vi "Documentation Panel.vi"() -> ()   [LabVIEW 2019, in "Panther Dashboard.lvlib"]
uses:
  Panther Dashboard.lvlib
panel:
  in  "Edit Module Description":bool caption="Module Description- Edit"
  in  "Module Description":string
  in  "Edit VI":bool caption="Event Connector Pane- Edit"
  out "Event Connector Pane":picture
  in  "Event Description":string
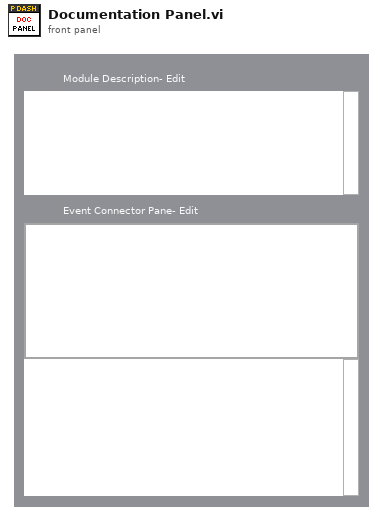
[diagram p1: front panel]
types:
  T1 = typedef "Panther Dashboard.lvlib/Broadcast Events--cluster.ctl" = cluster{"Module Did Init":refnum<user-event>, "Status Updated":refnum<user-event>, "Error Reported":refnum<user-event>, "Module Did Stop":refnum<user-event>, "Update Module Execution Status":refnum<user-event>, "References Updated":refnum<user-event>, "Projects Updated":refnum<user-event>, "Targets Updated":refnum<user-event>, "Progress updated":refnum<user-event>, "Scale Updated":refnum<user-event>, "Connector Pane Updated":refnum<user-event>, "Documentation Updated":refnum<user-event>, "Module Type Updated":refnum<user-event>, "Theme Updated":refnum<user-event>, "Panel Position Updated":refnum<user-event>}
  T2 = enum8{"Enabled", "Disabled", "Disabled and Grayed Out"}
  T3 = typedef "Panther Dashboard.lvlib/Documentation--cluster.ctl" = cluster{"Module Description":string, "Event Description":string}
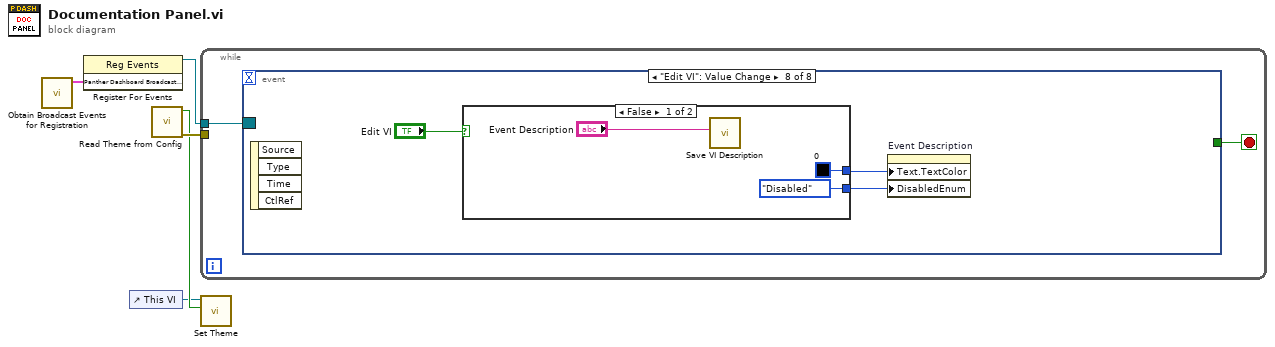
[diagram p0: block diagram]
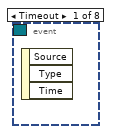
[diagram p2: hidden frame]
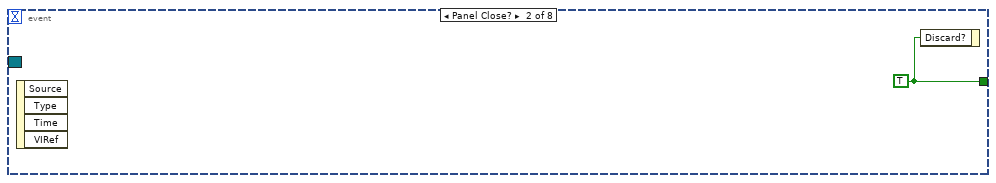
[diagram p3: hidden frame]
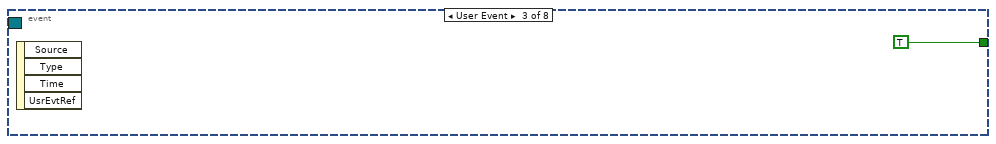
[diagram p4: hidden frame]
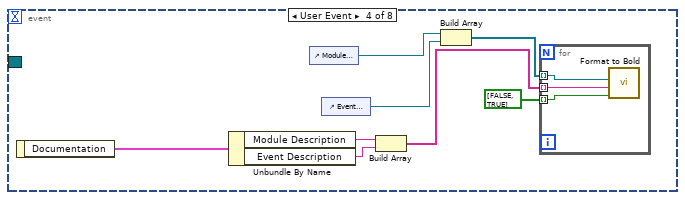
[diagram p5: hidden frame]
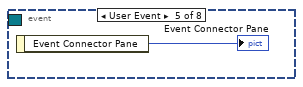
[diagram p6: hidden frame]
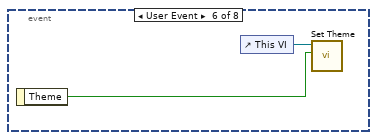
[diagram p7: hidden frame]
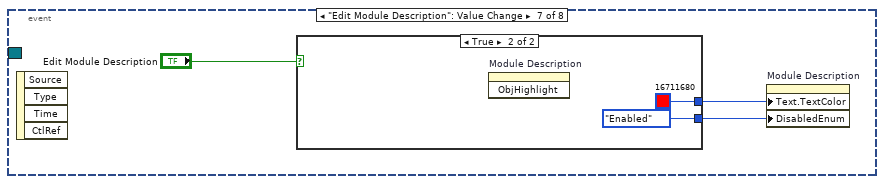
[diagram p8: hidden frame]
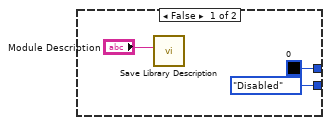
[diagram p9: hidden frame]
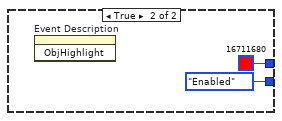
[diagram p10: hidden frame]
diagram:
  n1 = call "Obtain Broadcast Events for Registration.vi"() -> ("Panther Dashboard Broadcast Events"=w4:T1)  [unwired: 9 in, 2 out]
  n2 = register-events(w4) -> (reference out=w3:refnum<event-registration>)  [unwired: 2 in, 1 out]
  n3 = control-ref of="This VI"() -> (w1:refnum<vi>)
  n4 = call "Read Theme from Config.vi"() -> ("error out"=w5:errorcluster, "Theme"=w2:bool)  [unwired: 10 in]
  n5 = while {
    tunnel: w3 -> [w7]
    tunnel: w5 -> [_]
    stop <- w6 stop-if-true
    n6 = event shown="[7] \"Edit VI\": Value Change" {
      selector: w7 -> [_ _ _ _ _ _ _ _]
      dyn-events: _ -> [_ _ _ _ _ _ _ _]
      timeout: _ -> [_ _ _ _ _ _ _ _]
      tunnel: [_ w8 TRUE ("Discard?") _ _ _ _ _] -> w6
      event Timeout {
        n7 = event-data() -> ()  [unwired: 1 in, 3 out]
      }
      event Panel Close? {
        w8 = TRUE ("Discard?")
        n8 = event-data() -> ()  [unwired: 1 in, 4 out]
        n9 = event-data("Discard?"=w8) -> ()  [unwired: 1 in, 1 out]
      }
      event User Event {
        n10 = event-data() -> ()  [unwired: 1 in, 4 out]
      }
      event User Event {
        n11 = event-data() -> ("Documentation"=w10:T3)  [unwired: 1 in]
        n12 = Unbundle By Name(w10) -> ("Module Description"=w12:string, "Event Description"=w13:string)
        n13 = control-ref of="Module Description"() -> (w14:refnum<vi>)
        n14 = control-ref of="Event Description"() -> (w15:refnum<vi>)
        n15 = Build Array(w12, w13) -> (w17:string[])
        n16 = Build Array(w14, w15) -> (w16:refnum<vi>[])
        n17 = for {
          tunnel: w16 -> [w20] mode=indexing
          tunnel: w17 -> [w19] mode=indexing
          tunnel: bool[] [FALSE, TRUE] ("Adjust Height?") -> [w18] mode=indexing
          n18 = call "Format to Bold.vi"("Adjust Height?"=w18, "String Value"=w19, "String Ref"=w20) -> ()  [unwired: 9 in]
        }
      }
      event User Event {
        n19 = event-data() -> ("Event Connector Pane"=→"Event Connector Pane":picture)  [unwired: 1 in]
      }
      event User Event {
        n20 = event-data() -> ("Theme"=w22:bool)  [unwired: 1 in]
        n21 = control-ref of="This VI"() -> (w23:refnum<vi>)
        n22 = call "Set Theme.vi"("Dark?"=w22, "VI in"=w23) -> ()  [unwired: 10 in]
      }
      event "Edit Module Description": Value Change {
        n23 = event-data() -> ()  [unwired: 1 in, 4 out]
        n24 = case shown="True" "Edit Module Description" {
          tunnel: [u32 0 u32 16711680] -> w25
          tunnel: [T2."Disabled" ("Disabled") T2."Enabled" ("Disabled")] -> w24
          frame False {
            n25 = call "Save Library Description.vi"("Library Description"="Module Description") -> ()  [unwired: 10 in, 1 out]
          }
          frame True {
            n26 = invoke on="Module Description" class="Str" method="ObjHighlight"() -> ()  [unwired: 3 in, 3 out]
          }
        }
        n27 = property on="Module Description" class="Str"("Text.TextColor"=w25, "DisabledEnum"=w24) -> ()  [unwired: 2 in, 2 out]
      }
      event "Edit VI": Value Change {
        n28 = event-data() -> ()  [unwired: 1 in, 4 out]
        n29 = case shown="False" "Edit VI" {
          tunnel: [u32 0 u32 16711680] -> w33
          tunnel: [T2."Disabled" ("Disabled") T2."Enabled" ("Disabled")] -> w32
          frame False {
            n30 = call "Save VI Description.vi"("VI Description"="Event Description") -> ()  [unwired: 10 in, 1 out]
          }
          frame True {
            n31 = invoke on="Event Description" class="Str" method="ObjHighlight"() -> ()  [unwired: 3 in, 3 out]
          }
        }
        n32 = property on="Event Description" class="Str"("Text.TextColor"=w33, "DisabledEnum"=w32) -> ()  [unwired: 2 in, 2 out]
      }
    }
  }
  n33 = call "Set Theme.vi"("Dark?"=w2, "VI in"=w1) -> ()  [unwired: 10 in]
